vi "Write INIndex.vi"(8 "error in (no error)":errorcluster, 10 "INIndex":i32, 11 "BarcodeScan in":refnum<class "BarcodeScan.lvclass">) -> (0 "error out":errorcluster, 3 "BarcodeScan out":refnum<class "BarcodeScan.lvclass">)   [LabVIEW 2019, in "BarcodeScan.lvclass"]
uses:
  BarcodeScan.lvclass
  FlowIOCtrl.lvclass
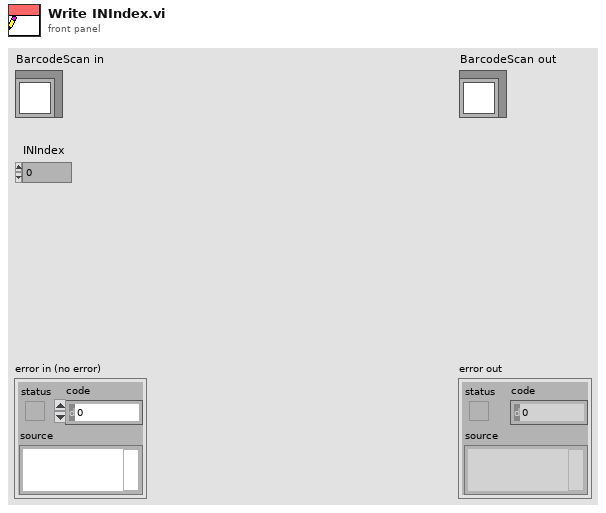
[diagram p1: front panel]
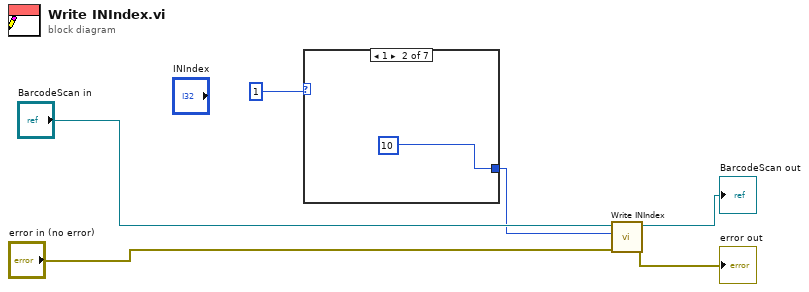
[diagram p0: block diagram]
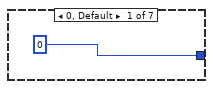
[diagram p2: hidden frame]
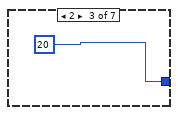
[diagram p3: hidden frame]
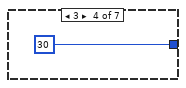
[diagram p4: hidden frame]
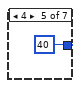
[diagram p5: hidden frame]
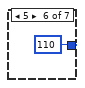
[diagram p6: hidden frame]
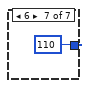
[diagram p7: hidden frame]
diagram:
  n1 = case shown="1" 1 {
    tunnel: [0 10 20 30 40 110 110 ("ModbusIOInput")] -> w2
    frame 0, Default {
    }
    frame 1 {
    }
    frame 2 {
    }
    frame 3 {
    }
    frame 4 {
    }
    frame 5 {
    }
    frame 6 {
    }
  }
  n2 = call-parent "Write INIndex.vi"("error in (no error)"="error in (no error)", "INIndex"=w2, "Station Action in"="BarcodeScan in") -> ("error out"=→"error out":errorcluster, "Station Action out"=→"BarcodeScan out":refnum<class "BarcodeScan.lvclass">)  [unwired: 7 in]
